vi "testFIFO.vi"() -> ()   [LabVIEW 2020]
uses:
  <vilib>/rvi/Emulation/niFpgaGetClockAttributes.vi
  <vilib>/rvi/Emulation/niFpgaSctlEmulationGetInTimedLoop.vi
  <vilib>/rvi/Emulation/niFpgaEmulationReportErrorSimple.vi
  <vilib>/rvi/interface/RandomDataEmulation/niFpgaRandomDataHandleErrors.vi
  <vilib>/rvi/Emulation/niFpgaCriticalErrorInLSC.vi
  <vilib>/rvi/DataTransferAndStorage/Container/XNode/niFpgaContainer.xnode
  <vilib>/rvi/interface/RandomDataEmulation/nirviRandomDataFpgaReadWriteTemplate.vi
panel:
  out "index":fxp<+,4,4>
  out "Array":u16[](array[numeric])
  out "LoopCount":i32
  out "FIFO Timeout\n2MTicks=50ms":i32=2000000
  in  "reset":bool
  out "Port Bits Only in U16":u16 format="%016b"
  out "Port# (1-4)":u8
  out "Parameter High Nibble Mid 4 bits  (xxNNNNxx xxxxxxxx)":u8 format="%04b"
  out "Low Byte (xxxxxxxx NNNNNNNN)":u8 format="%.0x"
  out "Element":u16=65535
  out "Request Type":T1(ring)
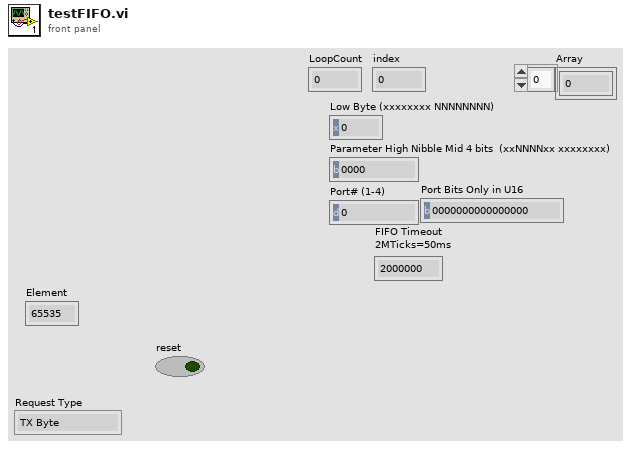
[diagram p1: front panel]
types:
  T1 = enum8{"TX Byte", "TX Clear", "Echo Request", "Parameter Change"}
  T2 = enum16{"TX Byte", "TX Clear", "Echo Request", "Parameter Change"}
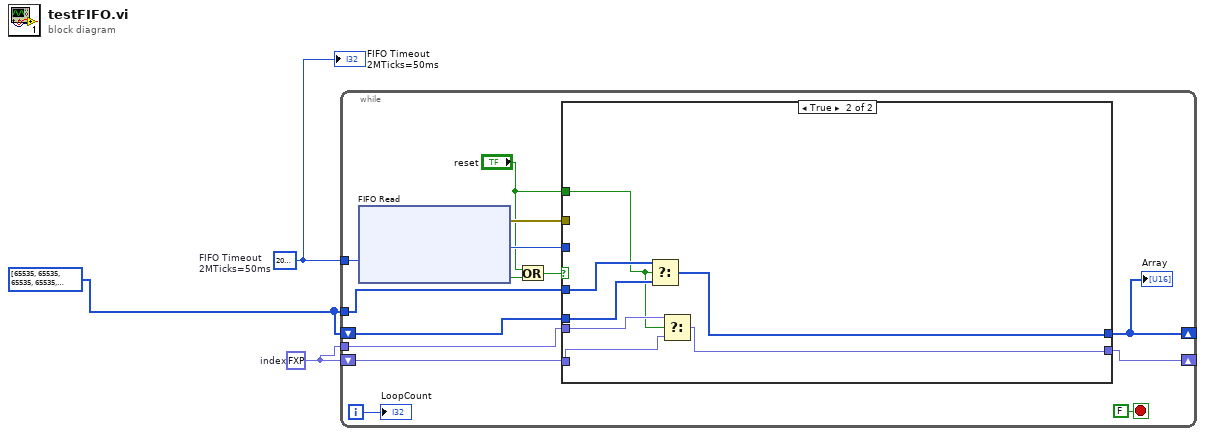
[diagram p0: block diagram]
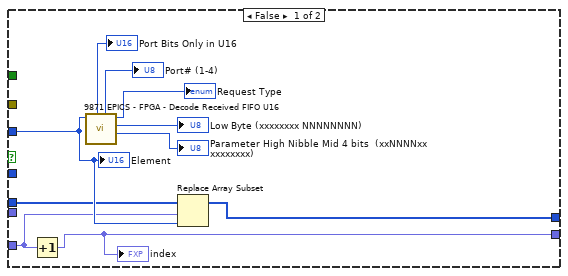
[diagram p2: hidden frame]
diagram:
  w2 = u16[] [65535, 65535, 65535, 65535, 65535, 65535, 65535, 65535, 65535, 65535, 65535, 65535, 65535, 65535, 65535, 65535]
  w1 = fxp<+,4,4> 0.0  # index
  w3 = 2000000  # FIFO Timeout 2MTicks=50ms
  n1 = while {
    tunnel: w3 -> [w14]
    shift-right: [w11] -> _
    shift-left: w1 -> [w13]
    tunnel: w2 -> [w9]
    shift-right: [w12] -> _
    shift-left: w2 -> [w10]
    tunnel: w1 -> [w8]
    i -> [w7]
    stop <- FALSE stop-if-true
    n2 = xnode ("FIFO Read")("Timeout"=w14) -> ("Element"=w15:u16, "Timed Out?"=w6:bool, "error out"=w16:errorcluster)  [unwired: 2 in, 1 out]
    n3 = Or(x="reset", y=w6) -> (x .or. y?=w5:bool)
    n4 = case shown="True" w5 {
      tunnel: w16 -> [_ _]
      tunnel: w15 -> [w22 _]
      tunnel: w13 -> [w19 w30]
      tunnel: w10 -> [w21 w33]
      tunnel: [w20 w32] -> w12
      tunnel: [w18 w29] -> w11
      tunnel: w9 -> [_ w34]
      tunnel: w8 -> [_ w31]
      tunnel: "reset" -> [_ w28]
      frame False {
        n5 = Increment(x=w19) -> (x+1=w18:fxp<+,4,4>)
        "index" <- w18
        n6 = call "9871 EPICS - FPGA - Decode Received FIFO U16.vi"("U16"=w22) -> ("Parameter High Nibble Mid 4 bits  (xxNNNNxx xxxxxxxx)"=→"Parameter High Nibble Mid 4 bits  (xxNNNNxx xxxxxxxx)":u8, "Low Byte (xxxxxxxx NNNNNNNN)"=→"Low Byte (xxxxxxxx NNNNNNNN)":u8, "Request Type"=→"Request Type":T2, "Port# (1-4)"=→"Port# (1-4)":u8, "Port Bits Only in U16"=→"Port Bits Only in U16":u16)  [unwired: 6 in]
        n7 = Replace Array Subset(array=w21, new element=w22, index=w19) -> (w20:u16[])
        "Element" <- w22
      }
      frame True {
        n8 = Select(t=w34, s=w28, f=w33) -> (s? t:f=w32:u16[])
        n9 = Select(t=w31, s=w28, f=w30) -> (s? t:f=w29:fxp<+,4,4>)
      }
    }
    "Array" <- w12
    "LoopCount" <- w7
  }
  "FIFO Timeout\n2MTicks=50ms" <- w3
